vi "扫描参数检查.vi"(7 "队列输入":refnum<queue>, 8 "NewVal输入":T1 {"测试参数"."反向极限电流(mA)" min=0.0 max=3000.0; "测试参数"."反向电压(V)" min=-40.0 max=40.0; "测试参数"."正向极限电流(mA)" min=0.0 max=3000.0; "测试参数"."正向电压(V)" min=-40.0 max=40.0; "时序参数"."反改变量(V)" min=0.0 max=40.0 step=5e-06; "时序参数"."正改变量(V)" min=0.0 max=40.0 step=5e-06; "时序参数"."nplc" min=0.001}, 11 "错误输入（无错误）":errorcluster) -> (0 "NewVal输出":T1 {"测试参数"."反向极限电流(mA)" min=0.0 max=3000.0; "测试参数"."反向电压(V)" min=-40.0 max=40.0; "测试参数"."正向极限电流(mA)" min=0.0 max=3000.0; "测试参数"."正向电压(V)" min=-40.0 max=40.0; "时序参数"."反改变量(V)" min=0.0 max=40.0 step=5e-06; "时序参数"."正改变量(V)" min=0.0 max=40.0 step=5e-06; "时序参数"."nplc" min=0.001}, 3 "错误输出":errorcluster)   [LabVIEW 2021]
uses:
  LabView Lib/QueueLib/QueueLib.lvlib
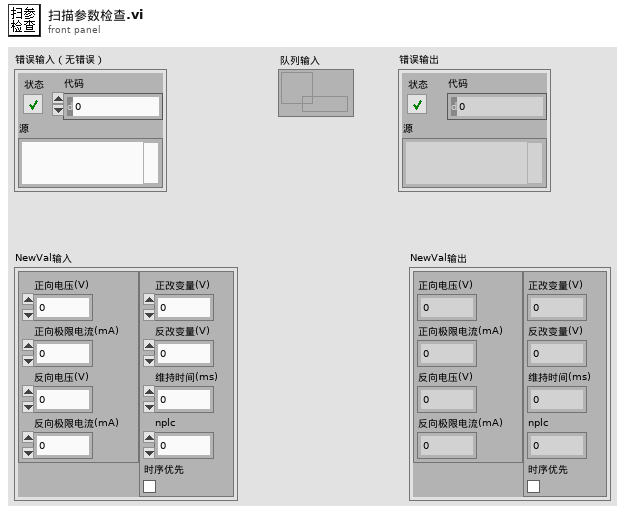
[diagram p1: front panel]
types:
  T1 = typedef "扫描参数.ctl" = cluster{"测试参数":cluster{"正向电压(V)":dbl, "正向极限电流(mA)":dbl, "反向电压(V)":dbl, "反向极限电流(mA)":dbl}, "时序参数":cluster{"正改变量(V)":dbl, "反改变量(V)":dbl, "维持时间(ms)":dbl, "nplc":dbl, "时序优先":bool}}
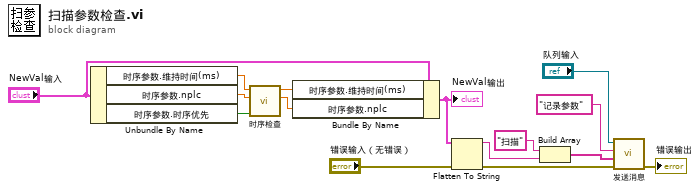
[diagram p0: block diagram]
diagram:
  n1 = Unbundle By Name("NewVal输入") -> ("时序参数.维持时间(ms)"=w2:dbl, "时序参数.nplc"=w3:dbl, "时序参数.时序优先"=w4:bool)
  n2 = call "时序检查.vi"("时序优先"=w4, "nplc"=w3, "测量间隔"=w2) -> ("nplc输出"=w6:dbl, "测量间隔输出"=w5:dbl)  [unwired: 7 in]
  n3 = Bundle By Name(cluster="NewVal输入", "时序参数.维持时间(ms)"=w5, "时序参数.nplc"=w6) -> (w15:T1)
  "NewVal输出" <- w15
  n4 = Flatten To String(anything=w15, error in (no error)="错误输入（无错误）") -> (data string=w11:string, error out=w7:errorcluster)  [unwired: 2 in, 1 out]
  n5 = Build Array("扫描" ("元素"), w11) -> (w13:string[])
  n6 = call-poly "发送消息.vi"("错误输入（无错误）"=w7, "数据"=w13, "消息"="记录参数", "输入队列"="队列输入") -> ("错误输出"=→"错误输出":errorcluster)  [unwired: 6 in, 1 out]
